vi "imp_test_v9_5.vi"() -> ()   [LabVIEW 2014]
uses:
  <vilib>/LabVIEW Targets/FPGA/cRIO/shared/nicrio_ModuleControls/nicrio_cRIO-9237_DataRatesRing.ctl
  <vilib>/LabVIEW Targets/FPGA/cRIO/shared/nicrio_ModuleControls/nicrio_cRIO-9237_ExcitationVoltageRing.ctl
  <vilib>/rvi/FXPMathLib/FxpSinAndCos/subVIs/nifxpmath_SinAndCos_SimConfig.ctl
  <vilib>/rvi/Emulation/niFpgaGetClockAttributes.vi
  <vilib>/rvi/Emulation/niFpgaSctlEmulationGetInTimedLoop.vi
  <vilib>/rvi/Emulation/niFpgaEmulationReportErrorSimple.vi
  <vilib>/rvi/Emulation/niFpgaProcessEmulError.vi
  <vilib>/rvi/interface/RandomDataEmulation/nirviRandomDataMultiElementFPGAFIFO.vi
  <instcachedir>/0/nirviRandomDataMultiElementFPGAFIFO_AD0CFC12EF974623A9C2E4184BC062B2.lvgen/nirviRandomDataMultiElementFPGAFIFO_AD0CFC12EF974623A9C2E4184BC062B2_025.vi
  <vilib>/rvi/interface/RandomDataEmulation/niFpgaRandomDataHandleErrors.vi
  <vilib>/rvi/Emulation/niFpgaCriticalErrorInLSC.vi
  <vilib>/rvi/FXPMathLib/FxpSinAndCos/simVIs/DllFxpSinAndCosTemp_sub.vi
  <vilib>/rvi/eio/common/nirviEmuTemplateMethod_errors.vi
  <vilib>/rvi/eio/common/nirviEmuTemplatePropertySet_errors.vi
  <vilib>/rvi/DataTransferAndStorage/Container/XNode/niFpgaContainer.xnode
  <vilib>/rvi/interface/RandomDataEmulation/nirviRandomDataFpgaMultiElementTemplate.vi
  <vilib>/rvi/FXPMathLib/FxpSinAndCos/XNode/nifxpmath_SinAndCos.xnode
  <vilib>/eio/EIONode/EIONode.xnode
  <vilib>/rvi/Analysis/measure/butterworth/XNode/niFpgaButterworthFilter.xnode
  <vilib>/eio/EIOPropertyNode/EIOPropertyNode.xnode
  <vilib>/rvi/eio/common/nirviEmuTemplatePropertyGet_errors.vi
  <vilib>/rvi/eio/common/nirviEmuTemplatePropertyGet_noerrors.vi
  <vilib>/rvi/eio/common/nirviEmuTemplatePropertySet_noerrors.vi
panel:
  in  "mt0_y2":u32
  in  "mt0_p2":u32
  out "Dy_d (Mavg w. f.)":fxp<+/-,36,14>
  out "Dp_d (Mavg w. f.)":fxp<+/-,36,14>
  in  "Dp_d (Mavg) coeff.":i32[](array[numeric])=[946630756, 63555534]
  in  "Dy_d (Mavg) coeff.":i32[](array[numeric])=[946630756, 63555534]
  out "omega_y (Mavg w. f.)":fxp<+/-,36,14>
  in  "omega_y(Mavg) coeff.":i32[](array[numeric])=[946630756, 63555534]
  out "omega_p (Mavg w. f)":fxp<+/-,36,14>
  in  "omega_P(Mavg) coeff.":i32[](array[numeric])=[946630756, 63555534]
  in  "FIFO":i16(ring) items=["Pitch_F+P", "imp ctrl", "Yaw_F+P"]
  out "PID (kHz)":fxp<+/-,20,10>
  in  "Set 6":bool
  in  "Set 5":bool
  in  "Set 4":bool
  in  "Set 3":bool
  in  "Set 2":bool
  in  "Set 1":bool
  out "Dy1_d (T)":fxp<+/-,36,13>
  out "omega_y1 (T)":fxp<+/-,36,13>
  out "Dp1_d (T)":fxp<+/-,36,13>
  out "omega_p1 (T)":fxp<+/-,36,13>
  out "Dy2_d (T)":fxp<+/-,36,13>
  out "Dp2_d (T)":fxp<+/-,36,13>
  out "omega_y2 (T)":fxp<+/-,36,13>
  out "omega_p2 (T)":fxp<+/-,36,13>
  out "mt_omega_y2":u32
  out "mt_omega_p2":u32
  out "rad_y2":fxp<+/-,33,20>
  out "D_y2":fxp<+/-,32,7>
  out "rad_y1":fxp<+/-,33,20>
  out "D_y1":fxp<+/-,32,7>
  out "Encoder Position_y1":i32
  out "Encoder Position_y2":i32
  out "Encoder Position_p2":i32
  out "D_p2":fxp<+/-,32,7>
  out "rad_p2":fxp<+/-,33,20>
  out "D_p1":fxp<+/-,32,7>
  out "rad_p1":fxp<+/-,33,20>
  out "Encoder Position_p1":i32
  in  "Mag. factor_y":fxp<+/-,20,3>
  in  "Mag. encoder_y":bool
  out "omega_y (rad/s)":fxp<+/-,36,13>
  out "Dy_d (mm/s)":fxp<+/-,36,13>
  in  "Vy. Est.":i16(ring) items=["T", "Mavg", "Mavg w. f."]
  out "omega_y (Mavg)":fxp<+/-,36,14>
  out "Dy_d (Mavg)":fxp<+/-,36,14>
  in  "Dy_d_M_avg_Tc (uSec)":i32
  out "Dp_d (Mavg)":fxp<+/-,36,14>
  out "omega_p (Mavg)":fxp<+/-,36,14>
  in  "Dp_d_M_avg_Tc (uSec)":i32
  out "Dp_d (T)":fxp<+/-,36,13>
  out "omega_p (T)":fxp<+/-,36,13>
  in  "Vp. Est.":i16(ring) items=["T", "Mavg", "Mavg w. f."]
  in  "Mag. factor_p":fxp<+/-,20,3>
  in  "Mag. encoder_p":bool
  in  "Belt_out_p":fxp<+/-,7,7>
  in  "Belt_in_p":fxp<+/-,6,6>
  in  "Belt_out_y":fxp<+/-,7,7>
  in  "Belt_in_y":fxp<+/-,6,6>
  out "Fp_dc":fxp<+/-,32,10>
  out "Fy_dc":fxp<+/-,32,10>
  in  "Zero_y":bool
  in  "Zero_p":bool
  in  "mt0_p1":u32
  in  "Encoder reset":bool
  in  "Dp_dd coeff.":i32[](array[numeric])=[946630756, 63555534]
  out "Dp_dd":fxp<+/-,36,25>
  out "dFp_PID":fxp<+/-,36,18>
  in  "dFp_PID coeff.":i32[](array[numeric])=[946630756, 63555534]
  out "fpt_i":fxp<+/-,34,18>
  in  "Kv_p":fxp<+/-,22,8>
  out "Dp_error":fxp<+/-,22,7>
  out "Dpr_sin":fxp<+/-,22,7>
  in  "Sin offset_p":fxp<+/-,22,7>
  in  "Sin magnitude_p":fxp<+/-,21,6>
  in  "Sin wave freq._p (Hz)":fxp<+/-,32,6>
  in  "Dpr_step":fxp<+/-,22,7>
  out "Dpr_for":fxp<+/-,22,7>
  in  "Command_p":i16(ring) items=["Step", "Sine"]
  in  "Ki_p":fxp<+/-,30,9>
  out "Fp_PID":fxp<+/-,36,16>
  in  "fp_tolorance":fxp<+,22,6>
  out "fp_tilde":fxp<+/-,33,10>
  in  "Kp_p":fxp<+/-,32,13>
  out "Fr_p":fxp<+/-,32,10>
  in  "S/F coeff_p":fxp<+/-,25,-10>
  in  "S/F coeff_y":fxp<+/-,25,-10>
  out "va_p":fxp<+/-,36,7>
  out "vb_p":fxp<+/-,37,8>
  out "vq_p_F":fxp<+/-,20,5> format="%.57g"
  out "vd_p_F":fxp<+/-,20,5>
  in  "Stop motor_p":bool
  out "Force_p":fxp<+/-,32,10>
  in  "Strain selection_p":i16(ring) items=["Raw", "Avg.8", "Avg.8 w. filter"]
  out "Strain_p (Avg8 w. f)":fxp<+/-,36,8>
  in  "Strain_p Avg.8 coeff.":i32[](array[numeric])=[946630756, 63555534]
  out "Strain_p (Avg8)":fxp<+/-,36,4>
  out "Raw Strain_p":fxp<+/-,36,4>
  out "Mod6/AI3":fxp<+/-,36,4>
  in  "Strain gage reset_p":bool
  out "Dp_d (mm/s)":fxp<+/-,36,13>
  out "omega_p (rad/s)":fxp<+/-,36,13>
  out "mt_omega_p1":u32
  out "rad_p(NrTheta)":fxp<+/-,33,20>
  out "D_p(mm)":fxp<+/-,32,7>
  out "Encoder Position_p":i32
  in  "Encoder reset_p":bool
  out "Strain_y (Avg8 w. f)":fxp<+/-,36,8>
  in  "Strain_y Avg8 coeff.":i32[](array[numeric])=[-898916953, 1957103773, 3888751]
  out "Dyr_for":fxp<+/-,22,7>
  in  "Command_y":i16(ring) items=["Step", "Sine"]
  out "Strain_y (Avg8)":fxp<+/-,36,4>
  in  "Strain selection_y":i16(ring) items=["Raw", "Avg.8", "Avg.8 w. filter"]
  out "vb_y":fxp<+/-,38,8>
  out "va_y":fxp<+/-,38,8>
  out "Fr_y":fxp<+/-,32,10>
  in  "Kv_y":fxp<+/-,22,8>
  out "Dy_error":fxp<+/-,22,7>
  out "Dyr_sin":fxp<+/-,22,7>
  in  "Sin offset_y":fxp<+/-,22,7>
  in  "Sin magnitude_y":fxp<+/-,21,6>
  out "Time now(s)":fxp<+,52,14>
  in  "Sin wave freq._y (Hz)":fxp<+/-,32,6>
  in  "Dyr_step":fxp<+/-,22,7>
  in  "Drive mode":i16(ring) items=["Backward", "Forward"]
  out "Dy_dd":fxp<+/-,36,25>
  in  "Dy_dd coeff.":i32[](array[numeric])=[946630756, 63555534]
  out "dFy_PID":fxp<+/-,36,18>
  in  "dFy_PID coeff.":i32[](array[numeric])=[946630756, 63555534]
  out "fyt_i":fxp<+/-,36,16>
  out "Fy_PID":fxp<+/-,36,16>
  in  "fy_tolorance":fxp<+,22,6>
  in  "Ki_y":fxp<+/-,30,9>
  out "fy_tilde":fxp<+/-,32,10>
  in  "Kp_y":fxp<+/-,32,13>
  out "vq_y_F":fxp<+/-,20,5> format="%.57g"
  out "vd_y_F":fxp<+/-,20,5>
  in  "Stop motor_y":bool
  out "Dy_d (T)":fxp<+/-,36,13>
  out "omega_y (T)":fxp<+/-,36,13>
  in  "mt0_y1":u32
  out "mt_omega_y1":u32
  out "rad_y(NrTheta)":fxp<+/-,33,20>
  out "D_y(mm)":fxp<+/-,32,7>
  out "Encoder Position_y":i32
  in  "Encoder reset_y":bool
  in  "Ini coe.":bool
  out "Loop rate (kHz)":fxp<+/-,36,7>
  out "Force_y":fxp<+/-,32,10>
  out "Raw Strain_y":fxp<+/-,36,4>
  in  "Strain gage reset_y":bool
  in  "Stop (Strain)":bool
  out "Mod6/AI2":fxp<+/-,36,4>
  in  "Excitation Voltage":T1 items=["2.5 Volts", "3.3 Volts", "5.0 Volts", "10.0 Volts", "External Excitation"]
  in  "Data Rate":T2=1 items=["50.000 kS/s (NI 9237)"=1, "25.000 kS/s (NI 9237)"=2, "16.667 kS/s (NI 9237)"=3, "12.500 kS/s (NI 9237)"=4, "10.000 kS/s (NI 9237)"=5, "8.333 kS/s (NI 9237)"=6, "7.143 kS/s (NI 9237)"=7, "6.250 kS/s (NI 9237)"=8, "5.556 kS/s (NI 9237)"=9, "5.000 kS/s (NI 9237)"=10, "4.545 kS/s (NI 9237)"=11, "4.167 kS/s (NI 9237)"=12, "3.846 kS/s (NI 9237)"=13, "3.571 kS/s (NI 9237)"=14, "3.333 kS/s (NI 9237)"=15, "3.125 kS/s (NI 9237)"=16, "2.941 kS/s (NI 9237)"=17, "2.778 kS/s (NI 9237)"=18, "2.632 kS/s (NI 9237)"=19, "2.500 kS/s (NI 9237)"=20, "2.381 kS/s (NI 9237)"=21, "2.273 kS/s (NI 9237)"=22, "2.174 kS/s (NI 9237)"=23, "2.083 kS/s (NI 9237)"=24, "2.000 kS/s (NI 9237)"=25, "1.923 kS/s (NI 9237)"=26, "1.852 kS/s (NI 9237)"=27, "1.786 kS/s (NI 9237)"=28, "1.724 kS/s (NI 9237)"=29, "1.667 kS/s (NI 9237)"=30, "1.613 kS/s (NI 9237)"=31]
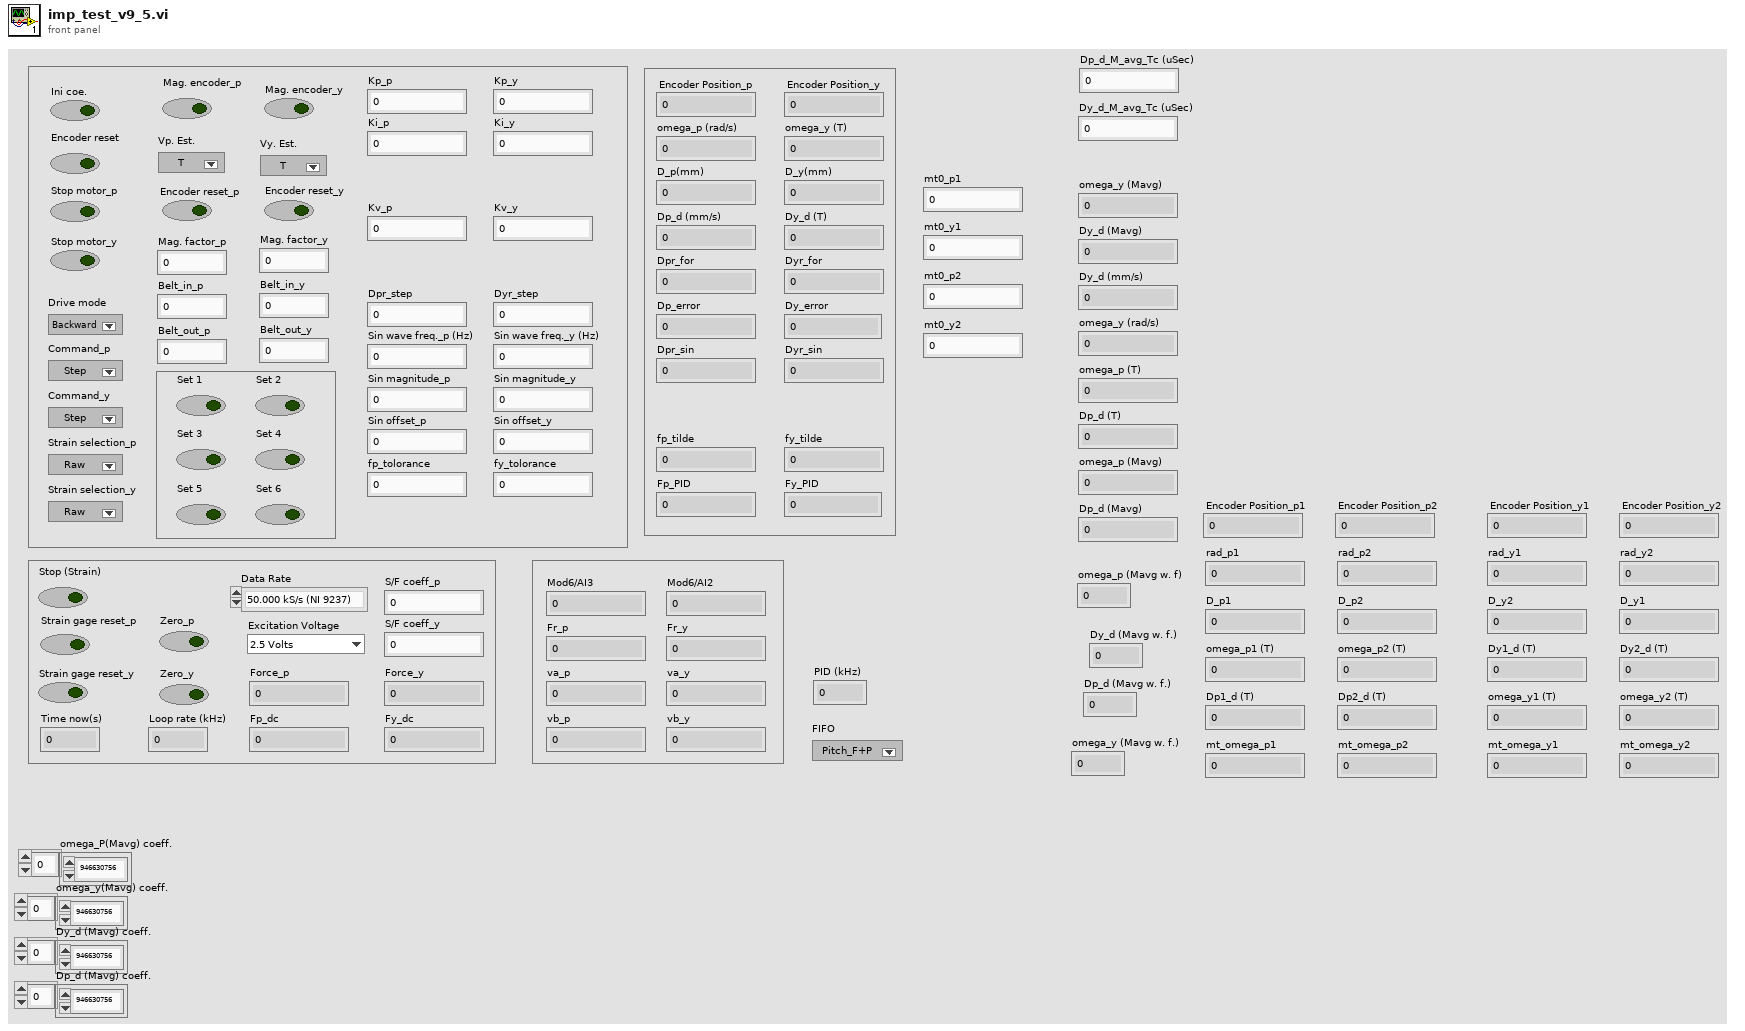
[diagram p1: front panel]
types:
  T1 = typedef "nicrio_cRIO-9237_ExcitationVoltageRing.ctl" = u8
  T2 = typedef "nicrio_cRIO-9237_DataRatesRing.ctl" = u8
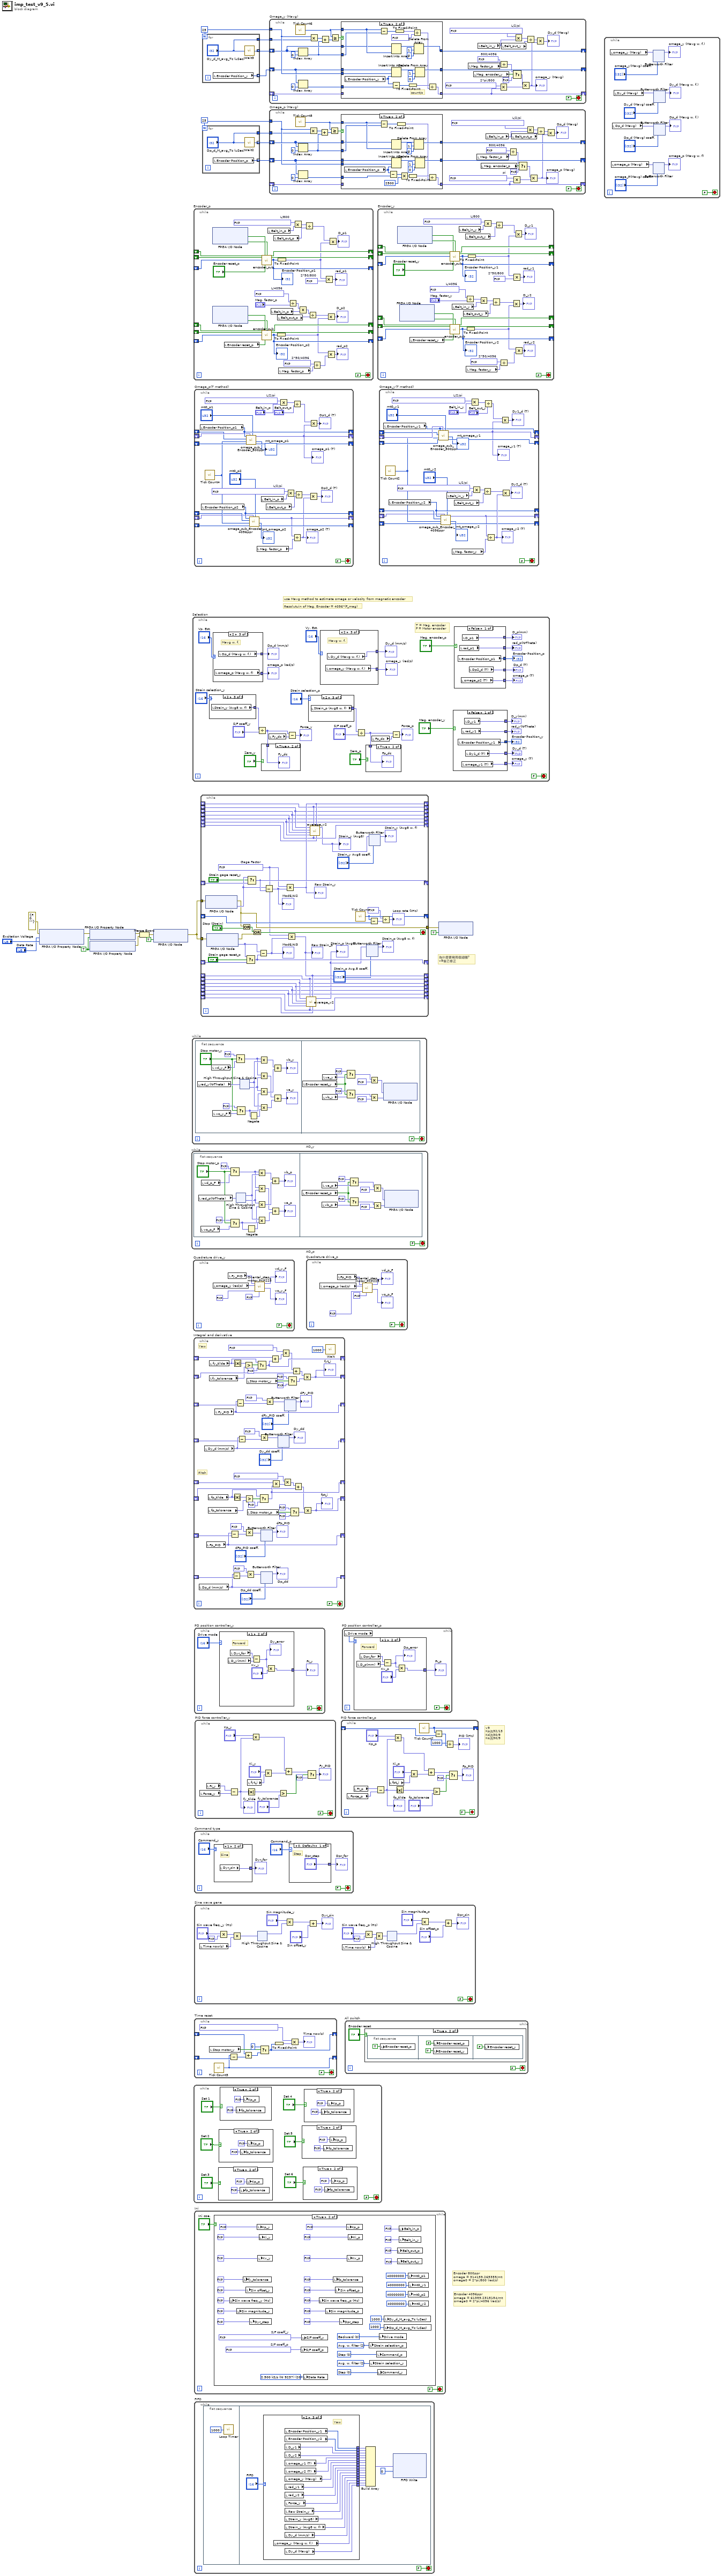
[diagram p0: block diagram]
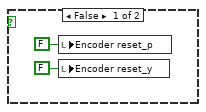
[diagram p10: hidden frame]
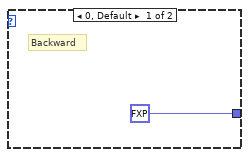
[diagram p11: hidden frame]
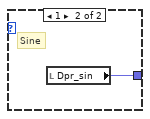
[diagram p12: hidden frame]
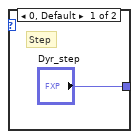
[diagram p13: hidden frame]
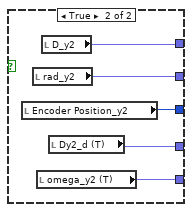
[diagram p14: hidden frame]
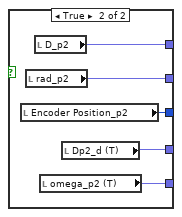
[diagram p15: hidden frame]
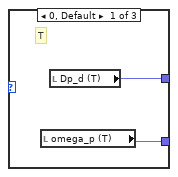
[diagram p16: hidden frame]
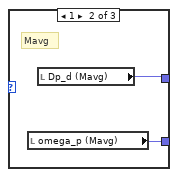
[diagram p17: hidden frame]
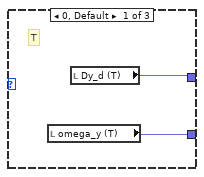
[diagram p18: hidden frame]
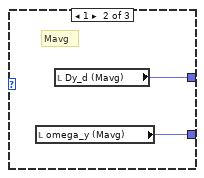
[diagram p19: hidden frame]
diagram:
  w5 = 25
  w8 = 25
  w13 = TRUE ("Half-Bridge Enable")
  # "Encoder 4096ppr\nomega = 61359.2315154/mt\nomega0 = 2*pi/4096 (rad/s)"
  # "Encoder 800ppr\nomega = 314159.265359/mt\nomega0 = 2*pi/800 (rad/s)"
  # "v9\nKp改32/13\nKd改30/9\nKo改30/9"
  # "Resolutuin of Mag. Encoder = 4096*(F_mag)"
  # "use Mavg method to estimate omega or velocity from magnetic encoder"
  # "為什麼要寫兩個迴圈?\nv9後已修正"
  n1 = xnode "FPGA I/O Property Node"("error in"=errorcluster {"status"=FALSE, "code"=0, "source"=""}, "Data Rate"="Data Rate", "Excitation Voltage"="Excitation Voltage") -> ("error out"=w18:errorcluster)  [unwired: 1 in, 1 out]
  n2 = xnode "FPGA I/O Property Node"("error in"=w18, "Half-Bridge Enable"=w13) -> ("error out"=w11:errorcluster)  [unwired: 1 in, 1 out]
  n3 = xnode "FPGA I/O Property Node"("Half-Bridge Enable"=w13) -> ("error out"=w10:errorcluster)  [unwired: 2 in, 1 out]
  n4 = Merge Errors(w11, w10) -> (w12:errorcluster)
  n5 = xnode "FPGA I/O Node"("error in"=w12, "Mod6/Start"=TRUE) -> ("error out"=w16:errorcluster)  [unwired: 1 in, 1 out]
  n6 = while "AO_p" {
    stop <- FALSE stop-if-true
    n7 = flat-sequence {
      frame #0 {
        n8 = local read "rad_p(NrTheta)"() -> (w33:fxp<+/-,33,20>)
        n9 = local read "vq_p_F"() -> (w34:fxp<+/-,20,5>)
        n10 = local read "vd_p_F"() -> (w36:fxp<+/-,20,5>)
        n11 = Select(t=fxp<+/-,20,5> 0.0, s="Stop motor_p", f=w36) -> (s? t:f=w25:fxp<+/-,20,5>)
        n12 = Select(t=fxp<+,1,1> 0.0, s="Stop motor_p", f=w34) -> (s? t:f=w24:fxp<+/-,20,5>)
        n13 = xnode "High Throughput Sine & Cosine"("x (pi)"=w33) -> ("sin(x)"=w27:fxp<+/-,16,2>, "cos(x)"=w26:fxp<+/-,16,2>)
        n14 = Negate(x=w24) -> (-x=w32:fxp<+/-,21,6>)
        n15 = Multiply(x=w25, y=w27) -> (x*y=w31:fxp<+/-,36,7>)
        n16 = Multiply(x=w25, y=w26) -> (x*y=w29:fxp<+/-,36,7>)
        n17 = Multiply(x=w26, y=w24) -> (x*y=w30:fxp<+/-,36,7>)
        n18 = Multiply(x=w27, y=w32) -> (x*y=w28:fxp<+/-,35,6>)
        n19 = Add(x=w31, y=w30) -> (x+y=→"vb_p":fxp<+/-,37,8>)
        n20 = Add(x=w29, y=w28) -> (x+y=→"va_p":fxp<+/-,36,7>)
      }
      frame #1 {
        n21 = local read "Encoder reset_p"() -> (w69:bool)
        n22 = local read "vb_p"() -> (w70:fxp<+/-,37,8>)
        n23 = local read "va_p"() -> (w71:fxp<+/-,36,7>)
        n24 = Select(t=fxp<+,2,2> 3.0, s=w69, f=w71) -> (s? t:f=w77:fxp<+/-,36,7>)
        n25 = Select(t=fxp<+,1,1> 0.0, s=w69, f=w70) -> (s? t:f=w76:fxp<+/-,37,8>)
        n26 = Multiply(x=w77, y=fxp<+/-,1,0> -0.5) -> (x*y=w72:fxp<+/-,36,6>)
        n27 = Multiply(x=w76, y=fxp<+/-,1,0> -0.5) -> (x*y=w73:fxp<+/-,36,6>)
        n28 = xnode "FPGA I/O Node"("Mod8/AO0"=w72, "Mod8/AO1"=w73) -> ()  [unwired: 2 in, 2 out]
      }
    }
  }
  n29 = while "AO_y" {
    stop <- FALSE stop-if-true
    n30 = flat-sequence {
      frame #0 {
        n31 = local read "rad_y(NrTheta)"() -> (w97:fxp<+/-,33,20>)
        n32 = local read "vd_y_F"() -> (w95:fxp<+/-,20,5>)
        n33 = local read "vq_y_F"() -> (w94:fxp<+/-,20,5>)
        n34 = Select(t=fxp<+/-,20,5> 0.0, s="Stop motor_y", f=w95) -> (s? t:f=w89:fxp<+/-,20,5>)
        n35 = Select(t=fxp<+/-,20,5> 0.0, s="Stop motor_y", f=w94) -> (s? t:f=w88:fxp<+/-,20,5>)
        n36 = xnode "High Throughput Sine & Cosine"("x (pi)"=w97) -> ("sin(x)"=w91:fxp<+/-,17,2>, "cos(x)"=w90:fxp<+/-,17,2>)
        n37 = Negate(x=w88) -> (-x=w87:fxp<+/-,21,6>)
        n38 = Multiply(x=w89, y=w91) -> (x*y=w86:fxp<+/-,37,7>)
        n39 = Multiply(x=w89, y=w90) -> (x*y=w84:fxp<+/-,37,7>)
        n40 = Multiply(x=w90, y=w88) -> (x*y=w85:fxp<+/-,37,7>)
        n41 = Multiply(x=w91, y=w87) -> (x*y=w83:fxp<+/-,36,6>)
        n42 = Add(x=w86, y=w85) -> (x+y=→"vb_y":fxp<+/-,38,8>)
        n43 = Add(x=w84, y=w83) -> (x+y=→"va_y":fxp<+/-,37,7>)
      }
      frame #1 {
        n44 = local read "Encoder reset_y"() -> (w130:bool)
        n45 = local read "va_y"() -> (w129:fxp<+/-,38,8>)
        n46 = local read "vb_y"() -> (w128:fxp<+/-,38,8>)
        n47 = Select(t=fxp<+,2,2> 3.0, s=w130, f=w129) -> (s? t:f=w134:fxp<+/-,38,8>)
        n48 = Select(t=fxp<+,1,1> 0.0, s=w130, f=w128) -> (s? t:f=w133:fxp<+/-,38,8>)
        n49 = Multiply(x=w134, y=fxp<+/-,1,0> -0.5) -> (x*y=w137:fxp<+/-,39,8>)
        n50 = Multiply(x=w133, y=fxp<+/-,1,0> -0.5) -> (x*y=w138:fxp<+/-,37,6>)
        n51 = xnode "FPGA I/O Node"("Mod8/AO2"=w137, "Mod8/AO3"=w138) -> ()  [unwired: 2 in, 2 out]
      }
    }
  }
  n52 = while "Selection" {
    stop <- FALSE stop-if-true
    # "T = Mag. encoder\nF = Motor encoder"
    n53 = case shown="2" "Strain selection_y" {
      tunnel: [w209 w210 w211] -> w170
      frame 0, Default {
        n54 = local read "Raw Strain_y"() -> (w209:fxp<+/-,36,4>)
      }
      frame 1 {
        n55 = local read "Strain_y (Avg8)"() -> (w210:fxp<+/-,36,4>)
      }
      frame 2 {
        n56 = local read "Strain_y (Avg8 w. f)"() -> (w211:fxp<+/-,36,8>)
      }
    }
    n57 = case shown="2" "Vp. Est." {
      tunnel: [w193 w194 w197] -> w153
      tunnel: [w192 w195 w196] -> w154
      frame 0, Default {
        # "T"
        n58 = local read "omega_p (T)"() -> (w193:fxp<+/-,36,13>)
        n59 = local read "Dp_d (T)"() -> (w192:fxp<+/-,36,13>)
      }
      frame 1 {
        # "Mavg"
        n60 = local read "omega_p (Mavg)"() -> (w194:fxp<+/-,36,14>)
        n61 = local read "Dp_d (Mavg)"() -> (w195:fxp<+/-,36,14>)
      }
      frame 2 {
        # "Mavg w. f."
        n62 = local read "omega_p (Mavg w. f)"() -> (w197:fxp<+/-,36,14>)
        n63 = local read "Dp_d (Mavg w. f.)"() -> (w196:fxp<+/-,36,14>)
      }
    }
    "Dp_d (mm/s)" <- w154
    "omega_p (rad/s)" <- w153
    n64 = Divide(x=w170, y="S/F coeff_y") -> (x/y=w163:fxp<+/-,32,10>)
    n65 = case shown="True" "Zero_y" {
      tunnel: w163 -> [_ w205]
      frame False {
      }
      frame True {
        "Fy_dc" <- w205
      }
    }
    n66 = local read "Fy_dc"() -> (w164:fxp<+/-,32,10>)
    n67 = Subtract(x=w163, y=w164) -> (x-y=→"Force_y":fxp<+/-,33,11>)
    n68 = case shown="2" "Strain selection_p" {
      tunnel: [w206 w207 w208] -> w168
      frame 0, Default {
        n69 = local read "Raw Strain_p"() -> (w206:fxp<+/-,36,4>)
      }
      frame 1 {
        n70 = local read "Strain_p (Avg8)"() -> (w207:fxp<+/-,36,4>)
      }
      frame 2 {
        n71 = local read "Strain_p (Avg8 w. f)"() -> (w208:fxp<+/-,36,8>)
      }
    }
    n72 = case shown="2" "Vy. Est." {
      tunnel: [w199 w201 w203] -> w156
      tunnel: [w198 w200 w202] -> w157
      frame 0, Default {
        # "T"
        n73 = local read "omega_y (T)"() -> (w198:fxp<+/-,36,13>)
        n74 = local read "Dy_d (T)"() -> (w199:fxp<+/-,36,13>)
      }
      frame 1 {
        # "Mavg"
        n75 = local read "omega_y (Mavg)"() -> (w200:fxp<+/-,36,14>)
        n76 = local read "Dy_d (Mavg)"() -> (w201:fxp<+/-,36,14>)
      }
      frame 2 {
        # "Mavg w. f."
        n77 = local read "omega_y (Mavg w. f.)"() -> (w202:fxp<+/-,36,14>)
        n78 = local read "Dy_d (Mavg w. f.)"() -> (w203:fxp<+/-,36,14>)
      }
    }
    "Dy_d (mm/s)" <- w156
    "omega_y (rad/s)" <- w157
    n79 = Divide(x=w168, y="S/F coeff_p") -> (x/y=w160:fxp<+/-,32,10>)
    n80 = case shown="True" "Zero_p" {
      tunnel: w160 -> [_ w204]
      frame False {
      }
      frame True {
        "Fp_dc" <- w204
      }
    }
    n81 = local read "Fp_dc"() -> (w158:fxp<+/-,32,10>)
    n82 = Subtract(x=w160, y=w158) -> (x-y=→"Force_p":fxp<+/-,33,11>)
    n83 = case shown="False" "Mag. encoder_y" {
      tunnel: [w176 w180] -> w144
      tunnel: [w175 w181] -> w145
      tunnel: [w174 w179] -> w147
      tunnel: [w172 w178] -> w141
      tunnel: [w173 w177] -> w140
      frame False {
        n84 = local read "Encoder Position_y1"() -> (w174:i32)
        n85 = local read "rad_y1"() -> (w176:fxp<+/-,33,20>)
        n86 = local read "omega_y1 (T)"() -> (w172:fxp<+/-,36,13>)
        n87 = local read "D_y1"() -> (w175:fxp<+/-,32,7>)
        n88 = local read "Dy1_d (T)"() -> (w173:fxp<+/-,36,13>)
      }
      frame True {
        n89 = local read "Encoder Position_y2"() -> (w179:i32)
        n90 = local read "rad_y2"() -> (w180:fxp<+/-,33,20>)
        n91 = local read "omega_y2 (T)"() -> (w178:fxp<+/-,36,13>)
        n92 = local read "D_y2"() -> (w181:fxp<+/-,32,7>)
        n93 = local read "Dy2_d (T)"() -> (w177:fxp<+/-,36,13>)
      }
    }
    "D_y(mm)" <- w145
    "rad_y(NrTheta)" <- w144
    "Encoder Position_y" <- w147
    "Dy_d (T)" <- w140
    "omega_y (T)" <- w141
    n94 = case shown="False" "Mag. encoder_p" {
      tunnel: [w186 w191] -> w149
      tunnel: [w185 w190] -> w150
      tunnel: [w184 w189] -> w151
      tunnel: [w182 w188] -> w143
      tunnel: [w183 w187] -> w142
      frame False {
        n95 = local read "Encoder Position_p1"() -> (w184:i32)
        n96 = local read "rad_p1"() -> (w185:fxp<+/-,33,20>)
        n97 = local read "omega_p2 (T)"() -> (w182:fxp<+/-,36,13>)
        n98 = local read "D_p1"() -> (w186:fxp<+/-,32,7>)
        n99 = local read "Dp2_d (T)"() -> (w183:fxp<+/-,36,13>)
      }
      frame True {
        n100 = local read "Encoder Position_p2"() -> (w189:i32)
        n101 = local read "rad_p2"() -> (w190:fxp<+/-,33,20>)
        n102 = local read "D_p2"() -> (w191:fxp<+/-,32,7>)
        n103 = local read "omega_p2 (T)"() -> (w188:fxp<+/-,36,13>)
        n104 = local read "Dp2_d (T)"() -> (w187:fxp<+/-,36,13>)
      }
    }
    "D_p(mm)" <- w149
    "rad_p(NrTheta)" <- w150
    "Encoder Position_p" <- w151
    "Dp_d (T)" <- w142
    "omega_p (T)" <- w143
  }
  n105 = while "Quadrature drive_y" {
    stop <- FALSE stop-if-true
    n106 = local read "omega_y (rad/s)"() -> (w218:fxp<+/-,36,13>)
    n107 = local read "Fy_PID"() -> (w214:fxp<+/-,36,16>)
    n108 = call "Oriental_step_motor_PKP225.vi"("F_Threshold"=fxp<+,12,12> 10.0, "dFmr"=fxp<+,1,1> 0.0 ("f"), "omega"=w218, "Fmr"=w214) -> ("vq_F"=→"vq_y_F":fxp<+/-,20,5>, "vd_F"=→"vd_y_F":fxp<+/-,20,5>)  [unwired: 6 in]
  }
  n109 = while "Encoder_p" {
    shift-right: [w256] -> _
    shift-left: _ -> [w255]
    shift-right: [w257] -> _
    shift-left: _ -> [w254]
    shift-right: [w251] -> _
    shift-left: _ -> [w253]
    shift-right: [w242] -> _
    shift-left: _ -> [w241]
    shift-right: [w243] -> _
    shift-left: _ -> [w244]
    shift-right: [w238] -> _
    shift-left: _ -> [w239]
    stop <- FALSE stop-if-true
    w234 = fxp<+/-,20,-5> 0.00048828125  # L/4096
    w232 = fxp<+/-,16,1> 0.0244140625  # 2*50/4096
    w250 = fxp<+/-,20,-5> 0.002499997615814209  # L/800
    w224 = fxp<+/-,16,1> 0.125  # 2*50/800
    n110 = xnode "FPGA I/O Node"() -> ("Mod7/DIO0"=w259:bool, "Mod7/DIO1"=w258:bool)  [unwired: 2 in, 2 out]
    n111 = xnode "FPGA I/O Node"() -> ("Mod7/DIO4"=w246:bool, "Mod7/DIO5"=w245:bool)  [unwired: 2 in, 2 out]
    n112 = local read "Encoder reset_p"() -> (w240:bool)
    n113 = call "encoder_sub.vi"("A_pre"=w255, "B_pre"=w254, "Encoder Position_pre"=w253, "A input"=w259, "Encoder Position Reset"="Encoder reset_p", "B input"=w258) -> ("A"=w256:bool, "B"=w257:bool, "Encoder Position (Counts)"=w251:i32)  [unwired: 19 in]
    "Encoder Position_p1" <- w251
    n114 = call "encoder_sub.vi"("A_pre"=w241, "B_pre"=w244, "Encoder Position_pre"=w239, "A input"=w246, "Encoder Position Reset"=w240, "B input"=w245) -> ("A"=w242:bool, "B"=w243:bool, "Encoder Position (Counts)"=w238:i32)  [unwired: 19 in]
    "Encoder Position_p2" <- w238
    n115 = local read "Belt_in_p"() -> (w249:fxp<+/-,6,6>)
    n116 = local read "Belt_in_p"() -> (w235:fxp<+/-,6,6>)
    n117 = local read "Belt_out_p"() -> (w247:fxp<+/-,7,7>)
    n118 = To Fixed-Point(number=w238) -> (fixed-point=w220:fxp<+/-,32,32>)  [unwired: 1 in]
    n119 = To Fixed-Point(number=w251) -> (fixed-point=w225:fxp<+/-,32,32>)  [unwired: 1 in]
    n120 = local read "Belt_out_p"() -> (w237:fxp<+/-,7,7>)
    n121 = local read "Mag. factor_p"() -> (w231:fxp<+/-,20,3>)
    n122 = Divide(x=w234, y="Mag. factor_p") -> (x/y=w233:fxp<+/-,41,13>)
    n123 = Multiply(x=w250, y=w249) -> (x*y=w248:fxp<+/-,26,1>)
    n124 = Multiply(x=w233, y=w235) -> (x*y=w236:fxp<+/-,46,18>)
    n125 = Divide(x=w248, y=w247) -> (x/y=w227:fxp<+/-,33,1>)
    n126 = Divide(x=w236, y=w237) -> (x/y=w222:fxp<+/-,53,18>)
    n127 = Divide(x=w232, y=w231) -> (x/y=w219:fxp<+/-,32,1>)
    n128 = Multiply(x=w225, y=w224) -> (x*y=→"rad_p1":fxp<+/-,33,20>)
    n129 = Multiply(x=w222, y=w220) -> (x*y=→"D_p2":fxp<+/-,37,7>)
    n130 = Multiply(x=w220, y=w219) -> (x*y=→"rad_p2":fxp<+/-,33,20>)
    n131 = Multiply(x=w227, y=w225) -> (x*y=→"D_p1":fxp<+/-,32,7>)
  }
  n132 = while "Integral and derivative" {
    shift-right: [w315] -> _
    shift-left: _ -> [w314]
    shift-right: [w307] -> _
    shift-left: _ -> [w306]
    shift-right: [w317] -> _
    shift-left: _ -> [w318]
    shift-right: [w297] -> _
    shift-left: _ -> [w296]
    shift-right: [w283] -> _
    shift-left: _ -> [w286]
    shift-right: [w276] -> _
    shift-left: _ -> [w275]
    shift-right: [w270] -> _
    shift-left: _ -> [w269]
    shift-right: [w265] -> _
    shift-left: _ -> [w266]
    stop <- FALSE stop-if-true
    # "Pitch"
    # "Yaw"
    n133 = local read "Dp_d (mm/s)"() -> (w265:fxp<+/-,36,13>)
    n134 = local read "Dy_d (mm/s)"() -> (w297:fxp<+/-,36,13>)
    n135 = local read "Fp_PID"() -> (w270:fxp<+/-,36,16>)
    n136 = local read "fp_tilde"() -> (w287:fxp<+/-,33,10>)
    n137 = local read "fp_tolorance"() -> (w290:fxp<+,22,6>)
    n138 = local read "fy_tolorance"() -> (w293:fxp<+,22,6>)
    n139 = local read "fy_tilde"() -> (w319:fxp<+/-,32,10>)
    n140 = local read "Fy_PID"() -> (w317:fxp<+/-,36,16>)
    n141 = Subtract(x=w270, y=w269) -> (x-y=w274:fxp<+/-,37,17>)
    n142 = Subtract(x=w265, y=w266) -> (x-y=w267:fxp<+/-,37,14>)
    n143 = Absolute Value(x=w287) -> (abs(x)=w291:fxp<+,33,10>)
    n144 = Absolute Value(x=w319) -> (abs(x)=w321:fxp<+,32,10>)
    n145 = Subtract(x=w317, y=w318) -> (x-y=w305:fxp<+/-,37,17>)
    n146 = Subtract(x=w297, y=w296) -> (x-y=w299:fxp<+/-,36,11>)
    n147 = Greater?(x=w321, y=w293) -> (0:w322:bool)
    n148 = Greater?(x=w291, y=w290) -> (0:w289:bool)
    n149 = Multiply(x=fxp<+,7,10> 1000.0, y=w274) -> (x*y=w272:fxp<+/-,32,18>)
    n150 = Multiply(x=fxp<+,7,10> 1000.0, y=w267) -> (x*y=w263:fxp<+/-,36,21>)
    n151 = local read "Stop motor_y"() -> (w308:bool)
    n152 = local read "Stop motor_p"() -> (w278:bool)
    n153 = Select(t=w319, s=w322, f=fxp<+/-,33,11> 0.0) -> (s? t:f=w315:fxp<+/-,33,11>)
    n154 = Select(t=w287, s=w289, f=fxp<+,1,1> 0.0) -> (s? t:f=w283:fxp<+/-,33,10>)
    n155 = Multiply(x=fxp<+,7,10> 1000.0, y=w299) -> (x*y=w298:fxp<+/-,36,21>)
    n156 = xnode "Butterworth Filter"("input data"=w272, "scaled coefficients"="dFp_PID coeff.") -> ("output data"=→"dFp_PID":fxp<+/-,36,22>)  [unwired: 1 in]
    n157 = xnode "Butterworth Filter"("input data"=w263, "scaled coefficients"="Dp_dd coeff.") -> ("output data"=→"Dp_dd":fxp<+/-,36,25>)  [unwired: 1 in]
    n158 = Multiply(x=fxp<+,7,10> 1000.0, y=w305) -> (x*y=w302:fxp<+/-,32,18>)
    n159 = Add(x=w314, y=w315) -> (x+y=w320:fxp<+/-,34,12>)
    n160 = Multiply(x=w286, y=w283) -> (x*y=w285:fxp<+/-,34,12>)
    n161 = xnode "Butterworth Filter"("input data"=w298, "scaled coefficients"="Dy_dd coeff.") -> ("output data"=→"Dy_dd":fxp<+/-,36,25>)  [unwired: 1 in]
    n162 = Multiply(x=fxp<+/-,30,12> 0.000499725341796875, y=w320) -> (x*y=w313:fxp<+/-,34,10>)
    n163 = Multiply(x=fxp<+/-,30,12> 0.000499725341796875, y=w285) -> (x*y=w282:fxp<+/-,34,10>)
    n164 = xnode "Butterworth Filter"("input data"=w302, "scaled coefficients"="dFy_PID coeff.") -> ("output data"=→"dFy_PID":fxp<+/-,36,22>)  [unwired: 1 in]
    n165 = Select(t=fxp<+,1,1> 0.0, s=w308, f=fxp<+,1,1> 1.0) -> (s? t:f=w311:fxp<+,1,1>)
    n166 = Select(t=fxp<+,1,1> 0.0, s=w278, f=fxp<+,1,1> 1.0) -> (s? t:f=w280:fxp<+,1,1>)
    n167 = Add(x=w313, y=w306) -> (x+y=w312:fxp<+/-,36,16>)
    n168 = Add(x=w282, y=w275) -> (x+y=w281:fxp<+/-,36,16>)
    n169 = Multiply(x=w312, y=w311) -> (x*y=w307:fxp<+/-,34,18>)
    "fyt_i" <- w307
    n170 = Multiply(x=w281, y=w280) -> (x*y=w276:fxp<+/-,34,18>)
    "fpt_i" <- w276
    n171 = call "Wait"("Count(uSec)"=u32 1000) -> ()  [unwired: 1 out]
  }
  n172 = while {
    stop <- FALSE stop-if-true
    n173 = case shown="True" "Set 3" {
      frame False {
      }
      frame True {
        n174 = local write "fp_tolorance"(fxp<+,22,6> 3.0 ("fp_tolorance")) -> ()
        n175 = local write "Kp_p"(fxp<+/-,36,9> 100.0 ("Kp_p")) -> ()
      }
    }
    n176 = case shown="True" "Set 2" {
      frame False {
      }
      frame True {
        n177 = local write "fp_tolorance"(fxp<+,22,6> 1.5 ("fp_tolorance")) -> ()
        n178 = local write "Kp_p"(fxp<+/-,36,9> 50.0 ("Kp_p")) -> ()
      }
    }
    n179 = case shown="True" "Set 1" {
      frame False {
      }
      frame True {
        n180 = local write "fp_tolorance"(fxp<+,22,6> 3.0 ("fp_tolorance")) -> ()
        n181 = local write "Kp_p"(fxp<+/-,36,9> 50.0 ("Kp_p")) -> ()
      }
    }
    n182 = case shown="True" "Set 5" {
      frame False {
      }
      frame True {
        n183 = local write "fp_tolorance"(fxp<+,22,6> 3.0 ("fp_tolorance")) -> ()
        n184 = local write "Kp_p"(fxp<+/-,36,9> 150.0 ("Kp_p")) -> ()
      }
    }
    n185 = case shown="True" "Set 6" {
      frame False {
      }
      frame True {
        n186 = local write "fp_tolorance"(fxp<+,22,6> 1.5 ("fp_tolorance")) -> ()
        n187 = local write "Kp_p"(fxp<+/-,36,9> 150.0 ("Kp_p")) -> ()
      }
    }
    n188 = case shown="True" "Set 4" {
      frame False {
      }
      frame True {
        n189 = local write "fp_tolorance"(fxp<+,22,6> 1.5 ("fp_tolorance")) -> ()
        n190 = local write "Kp_p"(fxp<+/-,36,9> 100.0 ("Kp_p")) -> ()
      }
    }
  }
  n191 = while "Omega_p(T method)" {
    shift-right: [w406] -> _
    shift-left: _ -> [w404]
    shift-right: [w387] -> _
    shift-left: _ -> [w405]
    shift-right: [w402] -> _
    shift-left: _ -> [w403]
    shift-right: [w380] -> _
    shift-left: _ -> [w379]
    shift-right: [w375] -> _
    shift-left: _ -> [w377]
    shift-right: [w383] -> _
    shift-left: _ -> [w382]
    stop <- FALSE stop-if-true
    w394 = fxp<+/-,32,0> 0.3183098859153688  # L/2/pi
    w399 = fxp<+/-,32,0> 0.3183098859153688  # L/2/pi
    n192 = local read "Encoder Position_p1"() -> (w406:i32)
    n193 = local read "Encoder Position_p2"() -> (w380:i32)
    n194 = call "Tick Count4"() -> ("Tick Count(Ticks)"=w381:u32)
    n195 = call "omega_sub_Encoder_800ppr.vi"("mt0"="mt0_p1", "omega_pre"=w405, "ticks_m_pre"=w403, "ticks"=w381, "count_pre"=w404, "count"=w406) -> ("ticks_m"=w402:u32, "mt"=→"mt_omega_p1":u32, "omega"=w387:fxp<+/-,36,13>)  [unwired: 3 in]
    "omega_p1 (T)" <- w387
    n196 = call "omega_sub_Encoder_4096ppr.vi"("mt0"="mt0_p2", "omega_pre"=w377, "ticks_m_pre"=w382, "ticks"=w381, "count_pre"=w379, "count"=w380) -> ("ticks_m"=w383:u32, "mt"=→"mt_omega_p2":u32, "omega"=w375:fxp<+/-,20,9>)  [unwired: 3 in]
    n197 = local read "Mag. factor_p"() -> (w395:fxp<+/-,20,3>)
    n198 = local read "Belt_in_p"() -> (w392:fxp<+/-,6,6>)
    n199 = local read "Belt_out_p"() -> (w391:fxp<+/-,7,7>)
    n200 = Multiply(x=w399, y="Belt_in_p") -> (x*y=w397:fxp<+/-,38,6>)
    n201 = Multiply(x=w394, y=w392) -> (x*y=w393:fxp<+/-,38,6>)
    n202 = Divide(x=w397, y="Belt_out_p") -> (x/y=w388:fxp<+/-,20,1>)
    n203 = Divide(x=w375, y=w395) -> (x/y=w376:fxp<+/-,32,1>)
    "omega_p2 (T)" <- w376
    n204 = Divide(x=w393, y=w391) -> (x/y=w386:fxp<+/-,45,6>)
    n205 = Multiply(x=w386, y=w376) -> (x*y=→"Dp2_d (T)":fxp<+/-,36,13>)
    n206 = Multiply(x=w388, y=w387) -> (x*y=→"Dp1_d (T)":fxp<+/-,36,13>)
  }
  n207 = while "PD position controller_y" {
    stop <- FALSE stop-if-true
    n208 = case shown="1" "Drive mode" {
      tunnel: [fxp<+/-,62,19> 0.0 w411] -> w408
      frame 0, Default {
        # "Backward"
      }
      frame 1 {
        # "Forward"
        n209 = local read "D_y(mm)"() -> (w415:fxp<+/-,32,7>)
        n210 = local read "Dyr_for"() -> (w412:fxp<+/-,22,7>)
        n211 = Subtract(x=w412, y=w415) -> (x-y=w414:fxp<+/-,33,8>)
        "Dy_error" <- w414
        n212 = Multiply(x=w414, y="Kv_y") -> (x*y=w411:fxp<+/-,54,15>)
      }
    }
    "Fr_y" <- w408
  }
  n213 = while "Command type" {
    stop <- FALSE stop-if-true
    n214 = case shown="1" "Command_y" {
      tunnel: ["Dyr_step" w424] -> w419
      frame 0, Default {
        # "Step"
      }
      frame 1 {
        # "Sine"
        n215 = local read "Dyr_sin"() -> (w424:fxp<+/-,22,7>)
      }
    }
    "Dyr_for" <- w419
    n216 = case shown="0, Default" "Command_p" {
      tunnel: ["Dpr_step" w422] -> w417
      frame 0, Default {
        # "Step"
      }
      frame 1 {
        # "Sine"
        n217 = local read "Dpr_sin"() -> (w422:fxp<+/-,22,7>)
      }
    }
    "Dpr_for" <- w417
  }
  n218 = while "Sine wave gene" {
    stop <- FALSE stop-if-true
    n219 = local read "Time now(s)"() -> (w442:fxp<+,52,14>)
    n220 = Multiply(x="Sin wave freq._y (Hz)", y=fxp<+/-,10,3> 2.0) -> (x*y=w443:fxp<+/-,41,9>)
    n221 = Multiply(x=w443, y=w442) -> (x*y=w441:fxp<+/-,41,19>)
    n222 = xnode "High Throughput Sine & Cosine"("x (pi)"=w441) -> ("sin(x)"=w436:fxp<+/-,16,2>)  [unwired: 1 out]
    n223 = Multiply(x="Sin magnitude_y", y=w436) -> (x*y=w439:fxp<+/-,37,8>)
    n224 = Add(x=w439, y="Sin offset_y") -> (x+y=→"Dyr_sin":fxp<+/-,37,8>)
    n225 = local read "Time now(s)"() -> (w431:fxp<+,52,14>)
    n226 = Multiply(x="Sin wave freq._p (Hz)", y=fxp<+/-,10,3> 2.0) -> (x*y=w435:fxp<+/-,42,9>)
    n227 = Multiply(x=w435, y=w431) -> (x*y=w432:fxp<+/-,41,19>)
    n228 = xnode "High Throughput Sine & Cosine"("x (pi)"=w432) -> ("sin(x)"=w426:fxp<+/-,16,2>)  [unwired: 1 out]
    n229 = Multiply(x="Sin magnitude_p", y=w426) -> (x*y=w429:fxp<+/-,37,8>)
    n230 = Add(x=w429, y="Sin offset_p") -> (x+y=→"Dpr_sin":fxp<+/-,37,8>)
  }
  n231 = while "Time reset" {
    shift-right: [w515] -> _
    shift-left: _ -> [w516]
    shift-right: [w510] -> _
    shift-left: _ -> [w511]
    stop <- FALSE stop-if-true
    n232 = local read "Stop motor_y"() -> (w517:bool)
    n233 = call "Tick Count3"() -> ("Tick Count(uSec)"=w515:u32)
    n234 = Subtract(x=w515, y=w516) -> (x-y=w514:u32)
    n235 = Add(x=w511, y=w514) -> (x+y=w513:u32)
    n236 = Select(t=u32 0, s=w517, f=w513) -> (s? t:f=w510:u32)
    n237 = To Fixed-Point(number=w510) -> (fixed-point=w509:fxp<+,32,32>)  [unwired: 1 in]
    n238 = Multiply(x=fxp<+,20,-18> 1.0000003385357559e-06, y=w509) -> (x*y=→"Time now(s)":fxp<+,52,14>)
  }
  n239 = while "Ini" {
    stop <- FALSE stop-if-true
    n240 = case shown="True" "Ini coe." {
      frame False {
      }
      frame True {
        w525 = T2 20 items=["50.000 kS/s (NI 9237)"=1, "25.000 kS/s (NI 9237)"=2, "16.667 kS/s (NI 9237)"=3, "12.500 kS/s (NI 9237)"=4, "10.000 kS/s (NI 9237)"=5, "8.333 kS/s (NI 9237)"=6, "7.143 kS/s (NI 9237)"=7, "6.250 kS/s (NI 9237)"=8, "5.556 kS/s (NI 9237)"=9, "5.000 kS/s (NI 9237)"=10, "4.545 kS/s (NI 9237)"=11, "4.167 kS/s (NI 9237)"=12, "3.846 kS/s (NI 9237)"=13, "3.571 kS/s (NI 9237)"=14, "3.333 kS/s (NI 9237)"=15, "3.125 kS/s (NI 9237)"=16, "2.941 kS/s (NI 9237)"=17, "2.778 kS/s (NI 9237)"=18, "2.632 kS/s (NI 9237)"=19, "2.500 kS/s (NI 9237)"=20, "2.381 kS/s (NI 9237)"=21, "2.273 kS/s (NI 9237)"=22, "2.174 kS/s (NI 9237)"=23, "2.083 kS/s (NI 9237)"=24, "2.000 kS/s (NI 9237)"=25, "1.923 kS/s (NI 9237)"=26, "1.852 kS/s (NI 9237)"=27, "1.786 kS/s (NI 9237)"=28, "1.724 kS/s (NI 9237)"=29, "1.667 kS/s (NI 9237)"=30, "1.613 kS/s (NI 9237)"=31] ("Data Rate")
        w539 = i16 0 items=["Step", "Sine"] ("Command_p")
        w540 = i16 2 items=["Raw", "Avg.", "Avg. w. filter"] ("Strain selection_p")
        w541 = i16 0 items=["Step", "Sine"] ("Command_y")
        w542 = i16 2 items=["Raw", "Avg.", "Avg. w. filter"] ("Strain selection_y")
        w544 = fxp<+/-,25,-10> 5.851034075021744e-07  # S/F coeff_p
        w543 = fxp<+/-,25,-10> 1.0477961041033268e-06  # S/F coeff_y
        w549 = i16 0 items=["Backward", "Forward"] ("Drive mode")
        n241 = local write "Sin wave freq._y (Hz)"(fxp<+/-,32,6> 1.0 ("Sin wave freq. (Hz)")) -> ()
        n242 = local write "Sin magnitude_y"(fxp<+/-,22,7> 5.0 ("Sin magnitude")) -> ()
        n243 = local write "fy_tolorance"(fxp<+,22,6> 5.0 ("f_tolorance")) -> ()
        n244 = local write "Sin offset_y"(fxp<+/-,38,9> 0.0 ("Sin offset")) -> ()
        n245 = local write "Dyr_step"(fxp<+/-,22,7> 0.0 ("Dr")) -> ()
        n246 = local write "Kp_y"(fxp<+/-,36,9> 30.0 ("Kp")) -> ()
        n247 = local write "Kv_y"(fxp<+/-,22,8> 0.0 ("Kv")) -> ()
        n248 = local write "Ki_y"(fxp<+/-,36,9> 0.0 ("Ki")) -> ()
        n249 = local write "S/F coeff_p"(w544) -> ()
        n250 = local write "S/F coeff_y"(w543) -> ()
        n251 = local write "Data Rate"(w525) -> ()
        n252 = local write "Sin wave freq._p (Hz)"(fxp<+/-,32,6> 1.0 ("Sin wave freq._p (Hz)")) -> ()
        n253 = local write "Sin magnitude_p"(fxp<+/-,21,6> 5.0 ("Sin magnitude_p")) -> ()
        n254 = local write "fp_tolorance"(fxp<+,22,6> 5.0 ("fp_tolorance")) -> ()
        n255 = local write "Sin offset_p"(fxp<+/-,22,7> 0.0 ("Sin offset_p")) -> ()
        n256 = local write "Dpr_step"(fxp<+/-,22,7> 0.0 ("Dpr_step")) -> ()
        n257 = local write "Kp_p"(fxp<+/-,36,9> 30.0 ("Kp_p")) -> ()
        n258 = local write "Kv_p"(fxp<+/-,22,8> 0.0 ("Kv_p")) -> ()
        n259 = local write "Ki_p"(fxp<+/-,36,9> 0.0 ("Ki_p")) -> ()
        n260 = local write "Strain selection_p"(w540) -> ()
        n261 = local write "Strain selection_y"(w542) -> ()
        n262 = local write "Command_p"(w539) -> ()
        n263 = local write "Command_y"(w541) -> ()
        n264 = local write "Drive mode"(w549) -> ()
        n265 = local write "Dp_d_M_avg_Tc (uSec)"(u32 1000 ("D_d_M_avg_Tc (uSec)")) -> ()
        n266 = local write "Dy_d_M_avg_Tc (uSec)"(1000 ("Dy_d_M_avg_Tc (uSec)")) -> ()
        n267 = local write "Belt_out_p"(fxp<+/-,7,7> 36.0 ("Belt_op")) -> ()
        n268 = local write "Belt_out_y"(fxp<+/-,7,7> 22.0 ("Belt_oy")) -> ()
        n269 = local write "Belt_in_p"(fxp<+/-,6,6> 14.0 ("Belt_mp")) -> ()
        n270 = local write "Belt_in_y"(fxp<+/-,6,6> 16.0 ("Belt_my")) -> ()
        n271 = local write "mt0_p1"(u32 40000000 ("mt0_p1")) -> ()
        n272 = local write "mt0_p2"(u32 40000000 ("mt0_p2")) -> ()
        n273 = local write "mt0_y1"(u32 40000000 ("mt0_y1")) -> ()
        n274 = local write "mt0_y2"(u32 40000000 ("mt0_y2")) -> ()
      }
    }
  }
  n275 = while "FIFO" {
    stop <- FALSE stop-if-true
    n276 = flat-sequence {
      frame #0 {
        n277 = call "Loop Timer"("Count(uSec)"=u32 1000) -> ()  [unwired: 1 out]
      }
      frame #1 {
        n278 = case shown="2" "FIFO" {
          tunnel: [w590 w606 w622] -> w574
          tunnel: [w589 w605 w621] -> w573
          tunnel: [w588 w604 w620] -> w572
          tunnel: [w587 w603 w619] -> w571
          tunnel: [w584 w602 w616] -> w569
          tunnel: [w585 w601 w617] -> w568
          tunnel: [w586 w600 w618] -> w567
          tunnel: [w582 w599 w614] -> w566
          tunnel: [w581 w598 w613] -> w565
          tunnel: [w580 w597 w612] -> w564
          tunnel: [w579 w596 w611] -> w563
          tunnel: [w578 w595 w610] -> w562
          tunnel: [w577 w594 w609] -> w561
          tunnel: [w576 w593 w608] -> w560
          tunnel: [w575 fxp<+,1,1> 0.0 ("element") w607] -> w559
          tunnel: [w583 fxp<+,1,1> 0.0 w615] -> w557
          frame 0 {
            # "Pitch"
            n279 = local read "omega_p (Mavg w. f)"() -> (w576:fxp<+/-,36,14>)
            n280 = local read "Encoder Position_p1"() -> (w590:i32)
            n281 = local read "Encoder Position_p2"() -> (w589:i32)
            n282 = local read "D_p1"() -> (w588:fxp<+/-,32,7>)
            n283 = local read "D_p2"() -> (w587:fxp<+/-,32,7>)
            n284 = local read "omega_p1 (T)"() -> (w586:fxp<+/-,36,13>)
            n285 = local read "omega_p2 (T)"() -> (w585:fxp<+/-,36,13>)
            n286 = local read "omega_p (Mavg)"() -> (w584:fxp<+/-,36,14>)
            n287 = local read "rad_p1"() -> (w583:fxp<+/-,33,20>)
            n288 = local read "rad_p2"() -> (w582:fxp<+/-,33,20>)
            n289 = local read "Force_p"() -> (w581:fxp<+/-,32,10>)
            n290 = local read "Raw Strain_p"() -> (w580:fxp<+/-,36,4>)
            n291 = local read "Strain_p (Avg8)"() -> (w579:fxp<+/-,36,4>)
            n292 = local read "Strain_p (Avg8 w. f)"() -> (w578:fxp<+/-,36,8>)
            n293 = local read "Dp_d (mm/s)"() -> (w577:fxp<+/-,36,13>)
            n294 = local read "Dp_d (Mavg)"() -> (w575:fxp<+/-,36,14>)
          }
          frame 1, Default {
            # "imp ctrl"
            n295 = local read "D_y(mm)"() -> (w606:fxp<+/-,32,7>)
            n296 = local read "Raw Strain_y"() -> (w605:fxp<+/-,36,4>)
            n297 = local read "Strain_y (Avg8)"() -> (w604:fxp<+/-,36,4>)
            n298 = local read "Strain_y (Avg8 w. f)"() -> (w603:fxp<+/-,36,8>)
            n299 = local read "Force_y"() -> (w600:fxp<+/-,32,10>)
            n300 = local read "Dy_d (T)"() -> (w601:fxp<+/-,36,13>)
            n301 = local read "Fy_dc"() -> (w602:fxp<+/-,32,10>)
            n302 = local read "D_p(mm)"() -> (w599:fxp<+/-,32,7>)
            n303 = local read "Raw Strain_p"() -> (w598:fxp<+/-,36,4>)
            n304 = local read "Strain_p (Avg8)"() -> (w597:fxp<+/-,36,4>)
            n305 = local read "Strain_p (Avg8 w. f)"() -> (w596:fxp<+/-,36,8>)
            n306 = local read "Force_p"() -> (w595:fxp<+/-,32,10>)
            n307 = local read "Dp_d (mm/s)"() -> (w594:fxp<+/-,36,13>)
            n308 = local read "Fp_dc"() -> (w593:fxp<+/-,32,10>)
          }
          frame 2 {
            # "Yaw"
            n309 = local read "omega_y (Mavg w. f.)"() -> (w608:fxp<+/-,36,14>)
            n310 = local read "Encoder Position_y1"() -> (w622:i32)
            n311 = local read "Encoder Position_y2"() -> (w621:i32)
            n312 = local read "D_y1"() -> (w620:fxp<+/-,32,7>)
            n313 = local read "D_y2"() -> (w619:fxp<+/-,32,7>)
            n314 = local read "omega_y1 (T)"() -> (w618:fxp<+/-,36,13>)
            n315 = local read "omega_y2 (T)"() -> (w617:fxp<+/-,36,13>)
            n316 = local read "omega_y (Mavg)"() -> (w616:fxp<+/-,36,14>)
            n317 = local read "rad_y1"() -> (w615:fxp<+/-,33,20>)
            n318 = local read "rad_y2"() -> (w614:fxp<+/-,33,20>)
            n319 = local read "Force_y"() -> (w613:fxp<+/-,32,10>)
            n320 = local read "Raw Strain_y"() -> (w612:fxp<+/-,36,4>)
            n321 = local read "Strain_y (Avg8)"() -> (w611:fxp<+/-,36,4>)
            n322 = local read "Strain_y (Avg8 w. f)"() -> (w610:fxp<+/-,36,8>)
            n323 = local read "Dy_d (mm/s)"() -> (w609:fxp<+/-,36,13>)
            n324 = local read "Dy_d (Mavg)"() -> (w607:fxp<+/-,36,14>)
          }
        }
        n325 = Build Array(w574, w573, w572, w571, w567, w568, w569, w557, w566, w565, w564, w563, w562, w561, w560, w559) -> (w558:fxp<+/-,64,32>[])
        n326 = xnode ("FIFO Write")("Element"=w558, "Timeout"=0) -> ()  [unwired: 1 in, 2 out]
      }
    }
  }
  n327 = while "PID force controller_y" {
    stop <- FALSE stop-if-true
    n328 = local read "Force_y"() -> (w625:fxp<+/-,32,10>)
    n329 = local read "Fr_y"() -> (w626:fxp<+/-,32,10>)
    n330 = Subtract(x=w626, y=w625) -> (x-y=w624:fxp<+/-,33,11>)
    "fy_tilde" <- w624
    n331 = Absolute Value(x=w624) -> (abs(x)=w636:fxp<+,32,10>)
    n332 = local read "fyt_i"() -> (w629:fxp<+/-,36,16>)
    n333 = Multiply(x="Kp_y", y=w624) -> (x*y=w623:fxp<+/-,64,23>)
    n334 = Multiply(x="Ki_y", y=w629) -> (x*y=w628:fxp<+/-,64,25>)
    n335 = Greater?(x=w636, y="fy_tolorance") -> (0:w634:bool)
    n336 = Add(x=w623, y=w628) -> (x+y=w627:fxp<+/-,36,16>)
    n337 = Select(t=w627, s=w634, f=fxp<+/-,51,14> 0.0) -> (s? t:f=→"Fy_PID":fxp<+/-,53,16>)
  }
  n338 = while {
    tunnel: w16 -> [w682]
    tunnel: [w656] -> w9
    shift-right: [w680] -> _
    shift-left: _ -> [w681]
    shift-right: [w676] -> _
    shift-left: _ -> [w677]
    shift-right: [w671] -> _
    shift-left: _ -> [w670]
    shift-right: [w670] -> _
    shift-left: _ -> [w669]
    shift-right: [w669] -> _
    shift-left: _ -> [w668]
    shift-right: [w668] -> _
    shift-left: _ -> [w667]
    shift-right: [w667] -> _
    shift-left: _ -> [w666]
    shift-right: [w666] -> _
    shift-left: _ -> [w665]
    shift-right: [w665] -> _
    shift-left: _ -> [w664]
    tunnel: w16 -> [w660]
    shift-right: [w653] -> _
    shift-left: _ -> [w654]
    shift-right: [w649] -> _
    shift-left: _ -> [w648]
    shift-right: [w648] -> _
    shift-left: _ -> [w647]
    shift-right: [w647] -> _
    shift-left: _ -> [w646]
    shift-right: [w646] -> _
    shift-left: _ -> [w645]
    shift-right: [w645] -> _
    shift-left: _ -> [w644]
    shift-right: [w644] -> _
    shift-left: _ -> [w643]
    shift-right: [w643] -> _
    shift-left: _ -> [w642]
    stop <- w657 stop-if-true
    w651 = fxp<+,20,2> 2.115001678466797  # Gage Factor
    n339 = xnode "FPGA I/O Node"("error in"=w682) -> ("error out"=w656:errorcluster, "Mod6/AI2"=w678:fxp<+/-,24,-4>)  [unwired: 1 in, 1 out]
    n340 = xnode "FPGA I/O Node"("error in"=w660) -> ("error out"=w658:errorcluster, "Mod6/AI3"=w652:fxp<+/-,24,-4>)  [unwired: 1 in, 1 out]
    n341 = Or(x=w656, y="Stop (Strain)") -> (x .or. y?=w659:bool)
    n342 = Select(t=w652, s="Strain gage reset_p", f=w654) -> (s? t:f=w653:fxp<+/-,24,-4>)
    n343 = Select(t=w678, s="Strain gage reset_y", f=w681) -> (s? t:f=w680:fxp<+/-,24,-4>)
    n344 = Or(x=w659, y=w658) -> (x .or. y?=w657:bool)
    n345 = Subtract(x=w652, y=w653) -> (x-y=w650:fxp<+/-,30,-3>)
    "Mod6/AI3" <- w650
    n346 = Subtract(x=w678, y=w680) -> (x-y=w679:fxp<+/-,30,-3>)
    "Mod6/AI2" <- w679
    n347 = Multiply(x=w651, y=w679) -> (x*y=w671:fxp<+/-,41,6>)
    "Raw Strain_y" <- w671
    n348 = Multiply(x=w651, y=w650) -> (x*y=w649:fxp<+/-,50,-1>)
    "Raw Strain_p" <- w649
    n349 = call "average_v2.vi"("Numeric 8"=w642, "Numeric"=w649, "Numeric 7"=w643, "Numeric 2"=w648, "Numeric 6"=w644, "Numeric 5"=w645, "Numeric 4"=w646, "Numeric 3"=w647) -> ("Mean (8pt)"=w641:fxp<+/-,32,4>)  [unwired: 1 in, 2 out]
    "Strain_p (Avg8)" <- w641
    n350 = call "average_v2.vi"("Numeric 8"=w664, "Numeric"=w671, "Numeric 7"=w665, "Numeric 2"=w670, "Numeric 6"=w666, "Numeric 5"=w667, "Numeric 4"=w668, "Numeric 3"=w669) -> ("Mean (8pt)"=w663:fxp<+/-,32,4>)  [unwired: 1 in, 2 out]
    "Strain_y (Avg8)" <- w663
    n351 = call "Tick Count"() -> ("Tick Count(uSec)"=w676:u32)
    n352 = xnode "Butterworth Filter"("input data"=w641, "scaled coefficients"="Strain_p Avg.8 coeff.") -> ("output data"=→"Strain_p (Avg8 w. f)":fxp<+/-,36,8>)  [unwired: 1 in]
    n353 = xnode "Butterworth Filter"("input data"=w663, "scaled coefficients"="Strain_y Avg8 coeff.") -> ("output data"=→"Strain_y (Avg8 w. f)":fxp<+/-,32,4>)  [unwired: 1 in]
    n354 = Subtract(x=w676, y=w677) -> (x-y=w674:fxp<+/-,32,16>)
    n355 = Divide(x=fxp<+,7,10> 1000.0, y=w674) -> (x/y=→"Loop rate (kHz)":fxp<+/-,40,27>)
  }
  n356 = for {
    N: w5 -> [_]
    tunnel: [w701] -> w4 mode=indexing
    tunnel: [w700] -> w3 mode=indexing
    tunnel: ["Dy_d_M_avg_Tc (uSec)"] -> w2
    n357 = local read "Encoder Position_y"() -> (w700:i32)
    n358 = call "Wait3"("Count(uSec)"="Dy_d_M_avg_Tc (uSec)") -> ("Tick Count(uSec)"=w701:u32)
  }
  n359 = for {
    N: w8 -> [_]
    tunnel: ["Dp_d_M_avg_Tc (uSec)"] -> w1
    tunnel: [w703] -> w7 mode=indexing
    tunnel: [w702] -> w6 mode=indexing
    n360 = local read "Encoder Position_p"() -> (w702:i32)
    n361 = call "Wait2"("Count(uSec)"="Dp_d_M_avg_Tc (uSec)") -> ("Tick Count(uSec)"=w703:u32)
  }
  n362 = while "Omega_y (Mavg)" {
    tunnel: w5 -> [w728]
    shift-right: [w726] -> _
    shift-left: w4 -> [w731]
    shift-right: [w725] -> _
    shift-left: w3 -> [w727]
    shift-right: [w720] -> _
    shift-left: _ -> [w724]
    tunnel: w2 -> [w719]
    stop <- FALSE stop-if-true
    w707 = fxp<+/-,32,0> 0.3183098859153688  # L/2/pi
    w716 = fxp<+,32,0> 0.1953125  # 800/4096
    w722 = fxp<+/-,27,3> 0.007853984832763672  # 2*pi/800
    n363 = call "Tick Count6"() -> ("Tick Count(uSec)"=w732:u32)
    n364 = Index Array(array=w731, index=0) -> (element=w730:u32)
    n365 = Index Array(array=w727, index=0) -> (element=w729:i32)
    n366 = Multiply(x=w728, y=w719) -> (x*y=w734:i32)
    n367 = Add(x=w734, y=w730) -> (x+y=w733:u32)
    n368 = Greater Or Equal?(x=w732, y=w733) -> (x >= y?=w723:bool)
    n369 = case shown="True" w723 {
      tunnel: w732 -> [_ w755]
      tunnel: w728 -> [_ w752]
      tunnel: w731 -> [w739 w754]
      tunnel: w730 -> [_ w753]
      tunnel: w729 -> [_ w749]
      tunnel: w727 -> [w738 w751]
      tunnel: [w737 w747] -> w720
      tunnel: [w739 w746] -> w726
      tunnel: [w738 w745] -> w725
      tunnel: w724 -> [w737 _]
      frame False {
      }
      frame True {
        # "count/s"
        n370 = local read "Encoder Position_y"() -> (w748:i32)
        n371 = Subtract(x=w755, y=w753) -> (x-y=w756:u32)
        n372 = Insert Into Array(array=w754, new element=w755) -> (w758:u32[])  [unwired: 1 in]
        n373 = Subtract(x=w748, y=w749) -> (x-y=w743:i32)
        n374 = Insert Into Array(array=w751, index=w752, new element=w748) -> (w759:i32[])
        n375 = To Fixed-Point(number=w756) -> (fixed-point=w742:fxp<+,32,32>)  [unwired: 1 in]
        n376 = To Fixed-Point(number=w743) -> (fixed-point=w750:fxp<+/-,32,32>)  [unwired: 1 in]
        n377 = Divide(x=w742, y=fxp<+,32,32> 1000000.0) -> (x/y=w741:fxp<+/-,64,32>)
        n378 = Delete From Array(array=w758, length=1, index=0) -> (array with subset deleted=w746:u32[])  [unwired: 1 out]
        n379 = Delete From Array(array=w759, length=1, index=0) -> (array with subset deleted=w745:i32[])  [unwired: 1 out]
        n380 = Divide(x=w750, y=w741) -> (x/y=w747:fxp<+/-,56,22>)
      }
    }
    n381 = local read "Mag. factor_p"() -> (w715:fxp<+/-,20,3>)
    n382 = local read "Mag. encoder_y"() -> (w718:bool)
    n383 = local read "Belt_in_y"() -> (w709:fxp<+/-,6,6>)
    n384 = Multiply(x=w722, y=w720) -> (x*y=w712:fxp<+/-,64,25>)
    n385 = Divide(x=w716, y=w715) -> (x/y=w714:fxp<+/-,32,1>)
    n386 = local read "Belt_out_y"() -> (w710:fxp<+/-,7,7>)
    n387 = Select(t=w714, s=w718, f=fxp<+/-,2,2> 1.0) -> (s? t:f=w713:fxp<+/-,33,2>)
    n388 = Multiply(x=w707, y=w709) -> (x*y=w708:fxp<+/-,38,6>)
    n389 = Multiply(x=w713, y=w712) -> (x*y=w711:fxp<+/-,64,27>)
    "omega_y (Mavg)" <- w711
    n390 = Divide(x=w708, y=w710) -> (x/y=w706:fxp<+/-,45,6>)
    n391 = Multiply(x=w706, y=w711) -> (x*y=→"Dy_d (Mavg)":fxp<+/-,64,32>)
  }
  n392 = while "Omega_p (Mavg)" {
    tunnel: w8 -> [w785]
    shift-right: [w783] -> _
    shift-left: w7 -> [w788]
    shift-right: [w782] -> _
    shift-left: w6 -> [w784]
    shift-right: [w781] -> _
    shift-left: _ -> [w780]
    tunnel: w1 -> [w778]
    stop <- FALSE stop-if-true
    w767 = fxp<+/-,27,3> 3.1415926814079285  # pi
    w769 = fxp<+,32,0> 0.1953125  # 800/4096
    w766 = fxp<+/-,32,0> 0.3183098859153688  # L/2/pi
    n393 = call "Tick Count5"() -> ("Tick Count(uSec)"=w789:u32)
    n394 = Index Array(array=w788, index=0) -> (element=w787:u32)
    n395 = Index Array(array=w784, index=0) -> (element=w786:i32)
    n396 = Multiply(x=w785, y=w778) -> (x*y=w791:i32)
    n397 = Add(x=w791, y=w787) -> (x+y=w790:u32)
    n398 = Greater Or Equal?(x=w789, y=w790) -> (x >= y?=w779:bool)
    n399 = case shown="True" w779 {
      tunnel: w789 -> [_ w812]
      tunnel: w785 -> [_ w809]
      tunnel: w788 -> [w796 w811]
      tunnel: w787 -> [_ w810]
      tunnel: w786 -> [_ w806]
      tunnel: w784 -> [w795 w808]
      tunnel: [w794 w804] -> w781
      tunnel: [w796 w803] -> w783
      tunnel: [w795 w802] -> w782
      tunnel: w780 -> [w794 _]
      frame False {
      }
      frame True {
        n400 = local read "Encoder Position_p"() -> (w805:i32)
        n401 = Subtract(x=w812, y=w810) -> (x-y=w813:u32)
        n402 = Subtract(x=w805, y=w806) -> (x-y=w798:i32)
        n403 = Insert Into Array(array=w811, new element=w812) -> (w815:u32[])  [unwired: 1 in]
        n404 = Insert Into Array(array=w808, index=w809, new element=w805) -> (w816:i32[])
        n405 = To Fixed-Point(number=w813) -> (fixed-point=w800:fxp<+,32,32>)  [unwired: 1 in]
        n406 = Multiply(x=w798, y=2500) -> (x*y=w799:i32)
        n407 = To Fixed-Point(number=w799) -> (fixed-point=w807:fxp<+/-,32,32>)  [unwired: 1 in]
        n408 = Delete From Array(array=w815, length=1, index=0) -> (array with subset deleted=w803:u32[])  [unwired: 1 out]
        n409 = Delete From Array(array=w816, length=1, index=0) -> (array with subset deleted=w802:i32[])  [unwired: 1 out]
        n410 = Divide(x=w807, y=w800) -> (x/y=w804:fxp<+/-,56,22>)
      }
    }
    n411 = local read "Mag. factor_p"() -> (w770:fxp<+/-,20,3>)
    n412 = local read "Mag. encoder_p"() -> (w777:bool)
    n413 = local read "Belt_in_p"() -> (w774:fxp<+/-,6,6>)
    n414 = Divide(x=w769, y=w770) -> (x/y=w768:fxp<+/-,32,1>)
    n415 = local read "Belt_out_p"() -> (w773:fxp<+/-,7,7>)
    n416 = Multiply(x=w767, y=w781) -> (x*y=w775:fxp<+/-,64,25>)
    n417 = Select(t=w768, s=w777, f=fxp<+/-,2,2> 1.0) -> (s? t:f=w762:fxp<+/-,33,2>)
    n418 = Multiply(x=w766, y=w774) -> (x*y=w772:fxp<+/-,38,6>)
    n419 = Multiply(x=w762, y=w775) -> (x*y=w765:fxp<+/-,64,27>)
    "omega_p (Mavg)" <- w765
    n420 = Divide(x=w772, y=w773) -> (x/y=w764:fxp<+/-,45,6>)
    n421 = Multiply(x=w764, y=w765) -> (x*y=→"Dp_d (Mavg)":fxp<+/-,64,32>)
  }
  n422 = while "Quadrature drive_p" {
    stop <- FALSE stop-if-true
    n423 = local read "omega_p (rad/s)"() -> (w825:fxp<+/-,36,13>)
    n424 = local read "Fp_PID"() -> (w821:fxp<+/-,36,16>)
    n425 = call "Oriental_step_motor_PKP225.vi"("F_Threshold"=fxp<+,12,12> 10.0, "dFmr"=fxp<+,1,1> 0.0 ("f"), "omega"=w825, "Fmr"=w821) -> ("vq_F"=→"vq_p_F":fxp<+/-,20,5>, "vd_F"=→"vd_p_F":fxp<+/-,20,5>)  [unwired: 6 in]
  }
  n426 = while "PID force controller_p" {
    shift-right: [w831] -> _
    shift-left: _ -> [w830]
    stop <- FALSE stop-if-true
    n427 = local read "Force_p"() -> (w838:fxp<+/-,32,10>)
    n428 = local read "Fr_p"() -> (w839:fxp<+/-,32,10>)
    n429 = Subtract(x=w839, y=w838) -> (x-y=w836:fxp<+/-,33,11>)
    "fp_tilde" <- w836
    n430 = local read "fpt_i"() -> (w834:fxp<+/-,34,18>)
    n431 = Multiply(x="Kp_p", y=w836) -> (x*y=w826:fxp<+/-,64,23>)
    n432 = Absolute Value(x=w836) -> (abs(x)=w845:fxp<+,32,10>)
    n433 = Multiply(x="Ki_p", y=w834) -> (x*y=w833:fxp<+/-,64,27>)
    n434 = call "Tick Count7"() -> ("Tick Count(uSec)"=w831:u32)
    n435 = Add(x=w826, y=w833) -> (x+y=w832:fxp<+/-,36,16>)
    n436 = Greater?(x=w845, y="fp_tolorance") -> (0:w842:bool)
    n437 = Subtract(x=w831, y=w830) -> (x-y=w829:u32)
    n438 = Divide(x=u32 1000, y=w829) -> (x/y=→"PID (kHz)":fxp<+/-,20,7>)
    n439 = Select(t=w832, s=w842, f=fxp<+,1,1> 0.0) -> (s? t:f=→"Fp_PID":fxp<+/-,36,16>)
  }
  n440 = while "PD position controller_p" {
    stop <- FALSE stop-if-true
    n441 = local read "Drive mode"() -> (w848:i16)
    n442 = case shown="1" w848 {
      tunnel: [fxp<+/-,62,19> 0.0 w850] -> w847
      frame 0, Default {
        # "Backward"
      }
      frame 1 {
        # "Forward"
        n443 = local read "D_p(mm)"() -> (w854:fxp<+/-,32,7>)
        n444 = local read "Dpr_for"() -> (w853:fxp<+/-,22,7>)
        n445 = Subtract(x=w853, y=w854) -> (x-y=w852:fxp<+/-,24,8>)
        "Dp_error" <- w852
        n446 = Multiply(x=w852, y="Kv_p") -> (x*y=w850:fxp<+/-,34,16>)
      }
    }
    "Fr_p" <- w847
  }
  n447 = while "All switch" {
    stop <- FALSE stop-if-true
    n448 = case shown="True" "Encoder reset" {
      frame False {
        n449 = local write "Encoder reset_p"(FALSE ("Encoder reset_p")) -> ()
        n450 = local write "Encoder reset_y"(FALSE ("Encoder reset_y")) -> ()
      }
      frame True {
        n451 = flat-sequence {
          frame #0 {
            n452 = local write "Encoder reset_p"(TRUE ("Encoder reset_p")) -> ()
          }
          frame #1 {
            n453 = local write "Encoder reset_y"(TRUE ("Encoder reset_y")) -> ()
            n454 = local write "Encoder reset_p"(FALSE ("Encoder reset_p")) -> ()
          }
          frame #2 {
            n455 = local write "Encoder reset_y"(FALSE ("Encoder reset_y")) -> ()
          }
        }
      }
    }
  }
  n456 = while "Encoder_y" {
    shift-right: [w901] -> _
    shift-left: _ -> [w893]
    shift-right: [w900] -> _
    shift-left: _ -> [w892]
    shift-right: [w891] -> _
    shift-left: _ -> [w889]
    shift-right: [w897] -> _
    shift-left: _ -> [w894]
    shift-right: [w896] -> _
    shift-left: _ -> [w895]
    shift-right: [w890] -> _
    shift-left: _ -> [w888]
    stop <- FALSE stop-if-true
    w878 = fxp<+/-,16,1> 0.0244140625  # 2*50/4096
    w883 = fxp<+/-,20,-5> 0.00048828125  # L/4096
    w886 = fxp<+/-,20,-5> 0.002499997615814209  # L/800
    w868 = fxp<+/-,16,1> 0.125  # 2*50/800
    n457 = xnode "FPGA I/O Node"() -> ("Mod7/DIO2"=w902:bool, "Mod7/DIO3"=w903:bool)  [unwired: 2 in, 2 out]
    n458 = xnode "FPGA I/O Node"() -> ("Mod7/DIO6"=w899:bool, "Mod7/DIO7"=w898:bool)  [unwired: 2 in, 2 out]
    n459 = local read "Encoder reset_y"() -> (w873:bool)
    n460 = call "encoder_sub.vi"("A_pre"=w893, "B_pre"=w892, "Encoder Position_pre"=w889, "A input"=w902, "Encoder Position Reset"="Encoder reset_y", "B input"=w903) -> ("A"=w901:bool, "B"=w900:bool, "Encoder Position (Counts)"=w891:i32)  [unwired: 19 in]
    "Encoder Position_y1" <- w891
    n461 = call "encoder_sub.vi"("A_pre"=w894, "B_pre"=w895, "Encoder Position_pre"=w888, "A input"=w899, "Encoder Position Reset"=w873, "B input"=w898) -> ("A"=w897:bool, "B"=w896:bool, "Encoder Position (Counts)"=w890:i32)  [unwired: 19 in]
    "Encoder Position_y2" <- w890
    n462 = local read "Belt_in_y"() -> (w881:fxp<+/-,6,6>)
    n463 = local read "Belt_in_y"() -> (w885:fxp<+/-,6,6>)
    n464 = local read "Belt_out_y"() -> (w879:fxp<+/-,7,7>)
    n465 = Divide(x=w883, y="Mag. factor_y") -> (x/y=w882:fxp<+/-,41,13>)
    n466 = local read "Belt_out_y"() -> (w884:fxp<+/-,7,7>)
    n467 = To Fixed-Point(number=w890) -> (fixed-point=w865:fxp<+/-,32,32>)  [unwired: 1 in]
    n468 = local read "Mag. factor_y"() -> (w877:fxp<+/-,20,3>)
    n469 = To Fixed-Point(number=w891) -> (fixed-point=w869:fxp<+/-,32,32>)  [unwired: 1 in]
    n470 = Multiply(x=w882, y=w881) -> (x*y=w880:fxp<+/-,46,18>)
    n471 = Multiply(x=w886, y=w885) -> (x*y=w887:fxp<+/-,26,1>)
    n472 = Divide(x=w880, y=w879) -> (x/y=w867:fxp<+/-,53,18>)
    n473 = Divide(x=w887, y=w884) -> (x/y=w871:fxp<+/-,33,1>)
    n474 = Divide(x=w878, y=w877) -> (x/y=w864:fxp<+/-,32,1>)
    n475 = Multiply(x=w867, y=w865) -> (x*y=→"D_y2":fxp<+/-,37,7>)
    n476 = Multiply(x=w869, y=w868) -> (x*y=→"rad_y1":fxp<+/-,33,20>)
    n477 = Multiply(x=w871, y=w869) -> (x*y=→"D_y1":fxp<+/-,32,7>)
    n478 = Multiply(x=w865, y=w864) -> (x*y=→"rad_y2":fxp<+/-,33,20>)
  }
  n479 = while "Omega_y(T method)" {
    shift-right: [w929] -> _
    shift-left: _ -> [w930]
    shift-right: [w916] -> _
    shift-left: _ -> [w932]
    shift-right: [w934] -> _
    shift-left: _ -> [w935]
    shift-right: [w907] -> _
    shift-left: _ -> [w908]
    shift-right: [w905] -> _
    shift-left: _ -> [w904]
    shift-right: [w911] -> _
    shift-left: _ -> [w910]
    stop <- FALSE stop-if-true
    w923 = fxp<+/-,32,0> 0.3183098859153688  # L/2/pi
    w928 = fxp<+/-,32,0> 0.3183098859153688  # L/2/pi
    n480 = local read "Encoder Position_y1"() -> (w929:i32)
    n481 = call "Tick Count2"() -> ("Tick Count(Ticks)"=w909:u32)
    n482 = local read "Encoder Position_y2"() -> (w907:i32)
    n483 = call "omega_sub_Encoder_800ppr.vi"("mt0"="mt0_y1", "omega_pre"=w932, "ticks_m_pre"=w935, "ticks"=w909, "count_pre"=w930, "count"=w929) -> ("ticks_m"=w934:u32, "mt"=→"mt_omega_y1":u32, "omega"=w916:fxp<+/-,36,13>)  [unwired: 3 in]
    "omega_y1 (T)" <- w916
    n484 = call "omega_sub_Encoder_4096ppr.vi"("mt0"="mt0_y2", "omega_pre"=w904, "ticks_m_pre"=w910, "ticks"=w909, "count_pre"=w908, "count"=w907) -> ("ticks_m"=w911:u32, "mt"=→"mt_omega_y2":u32, "omega"=w905:fxp<+/-,20,9>)  [unwired: 3 in]
    n485 = local read "Belt_in_y"() -> (w922:fxp<+/-,6,6>)
    n486 = local read "Mag. factor_y"() -> (w924:fxp<+/-,20,3>)
    n487 = local read "Belt_out_y"() -> (w920:fxp<+/-,7,7>)
    n488 = Multiply(x=w928, y="Belt_in_y") -> (x*y=w926:fxp<+/-,38,6>)
    n489 = Multiply(x=w923, y=w922) -> (x*y=w921:fxp<+/-,38,6>)
    n490 = Divide(x=w921, y=w920) -> (x/y=w914:fxp<+/-,45,6>)
    n491 = Divide(x=w926, y="Belt_out_y") -> (x/y=w917:fxp<+/-,20,1>)
    n492 = Divide(x=w905, y=w924) -> (x/y=w913:fxp<+/-,32,1>)
    "omega_y2 (T)" <- w913
    n493 = Multiply(x=w917, y=w916) -> (x*y=→"Dy1_d (T)":fxp<+/-,36,13>)
    n494 = Multiply(x=w914, y=w913) -> (x*y=→"Dy2_d (T)":fxp<+/-,36,13>)
  }
  n495 = xnode "FPGA I/O Node"("error in"=w9, "Mod6/Stop"=TRUE) -> ()  [unwired: 1 in, 2 out]
  n496 = while {
    stop <- FALSE stop-if-true
    n497 = local read "omega_y (Mavg)"() -> (w944:fxp<+/-,36,14>)
    n498 = local read "omega_p (Mavg)"() -> (w948:fxp<+/-,36,14>)
    n499 = local read "Dp_d (Mavg)"() -> (w940:fxp<+/-,36,14>)
    n500 = local read "Dy_d (Mavg)"() -> (w941:fxp<+/-,36,14>)
    n501 = xnode "Butterworth Filter"("input data"=w944, "scaled coefficients"="omega_y(Mavg) coeff.") -> ("output data"=→"omega_y (Mavg w. f.)":fxp<+/-,36,18>)  [unwired: 1 in]
    n502 = xnode "Butterworth Filter"("input data"=w948, "scaled coefficients"="omega_P(Mavg) coeff.") -> ("output data"=→"omega_p (Mavg w. f)":fxp<+/-,36,18>)  [unwired: 1 in]
    n503 = xnode "Butterworth Filter"("input data"=w941, "scaled coefficients"="Dy_d (Mavg) coeff.") -> ("output data"=→"Dy_d (Mavg w. f.)":fxp<+/-,36,18>)  [unwired: 1 in]
    n504 = xnode "Butterworth Filter"("input data"=w940, "scaled coefficients"="Dp_d (Mavg) coeff.") -> ("output data"=→"Dp_d (Mavg w. f.)":fxp<+/-,36,18>)  [unwired: 1 in]
  }
